vi "Data Reference Interleave.vi"(10 "Data Symbols":cdb[](array[numeric]), 11 "Reference Symbols":cdb[](array[numeric])) -> (3 "Interleaved Output":cdb[](array[numeric]))   [LabVIEW 2022 SP3]
doc: "1. Inserts known refrence symbols\n2. Interleaves Symbols"
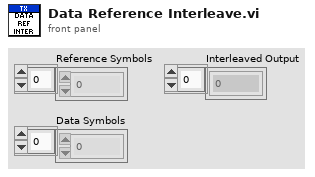
[diagram p1: front panel]
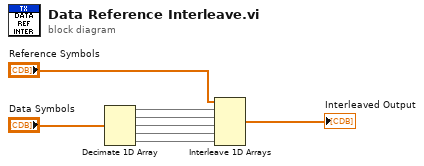
[diagram p0: block diagram]
diagram:
  n1 = Decimate 1D Array "Decimate 1D Array"("Data Symbols") -> (w1:cdb[], w2:cdb[], w3:cdb[], w4:cdb[], w5:cdb[])
  n2 = Interleave 1D Arrays "Interleave 1D Arrays"("Reference Symbols", w1, w2, w3, w4, w5) -> (→"Interleaved Output":cdb[])
